vi "Make bounding rectangle from center and sizes.vi"(3 "Y size":i32=21, 4 "Center (pix)":cluster{"X":i32, "Y":i32}={"X"=100, "Y"=200}, 5 "X size":i32=10) -> (1 "Bounding Rect":T1={"Left"=95.0, "Top"=190.0, "Right"=105.0, "Bottom"=211.0})   [LabVIEW 2013]
doc: "Creates bounding rectangle from center and and Y size."
uses:
  Project Vis/Image Analysis/Analysis type defs/Bounding rectangle cluster.ctl
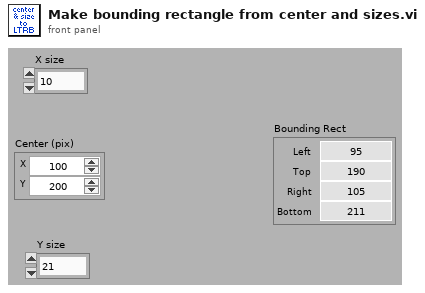
[diagram p1: front panel]
types:
  T1 = typedef "Bounding rectangle cluster.ctl" = cluster{"Left":dbl, "Top":dbl, "Right":dbl, "Bottom":dbl}
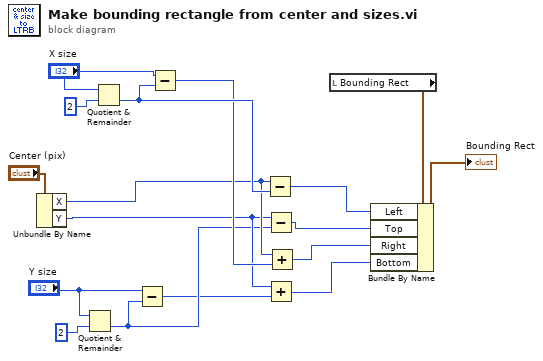
[diagram p0: block diagram]
diagram:
  n1 = Unbundle By Name("Center (pix)") -> ("X"=w5:i32, "Y"=w4:i32)
  n2 = Quotient & Remainder(x="Y size", y=2) -> (floor(x/y)=w2:i32)  [unwired: 1 out]
  n3 = Quotient & Remainder(x="X size", y=2) -> (floor(x/y)=w7:i32)  [unwired: 1 out]
  n4 = Subtract(x="Y size", y=w2) -> (x-y=w1:i32)
  n5 = Subtract(x="X size", y=w7) -> (x-y=w6:i32)
  n6 = Subtract(x=w5, y=w7) -> (x-y=w16:i32)
  n7 = Subtract(x=w4, y=w2) -> (x-y=w15:i32)
  n8 = Add(x=w4, y=w1) -> (x+y=w13:i32)
  n9 = Add(x=w5, y=w6) -> (x+y=w14:i32)
  n10 = local read "Bounding Rect"() -> (w12:T1)
  n11 = Bundle By Name(cluster=w12, "Left"=w16, "Top"=w15, "Right"=w14, "Bottom"=w13) -> (→"Bounding Rect":T1)
